vi "Z to circle.vi"(8 "Error In":errorcluster, 10 "Plot points":i32=90, 11 "Z":cdb[](array[numeric])) -> (0 "Error Out":errorcluster, 1 "y0":dbl, 2 "x0":dbl, 3 "plot":cluster{"Array":dbl[], "Array":dbl[]}, 4 "r":dbl format="%.2f", 5 "theta":dbl, 6 "Circle fit":cluster{"Array":dbl[], "Array":dbl[]}[](graph))   [LabVIEW 2016]
uses:
  <vilib>/gmath/NI_Gmath.lvlib
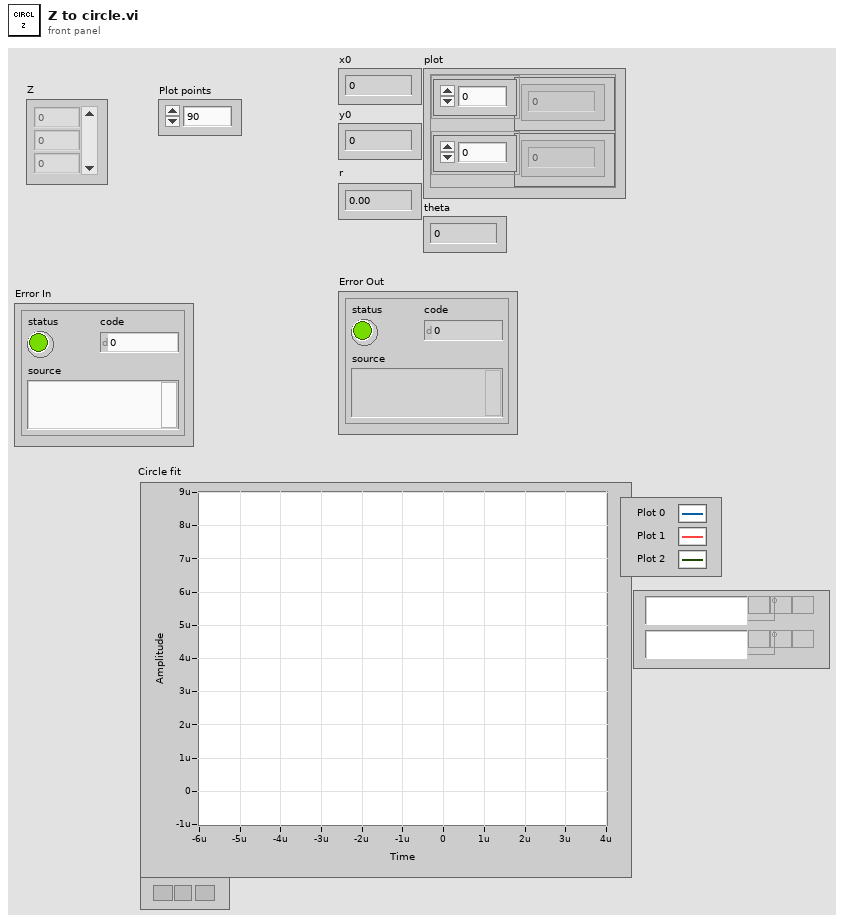
[diagram p1: front panel]
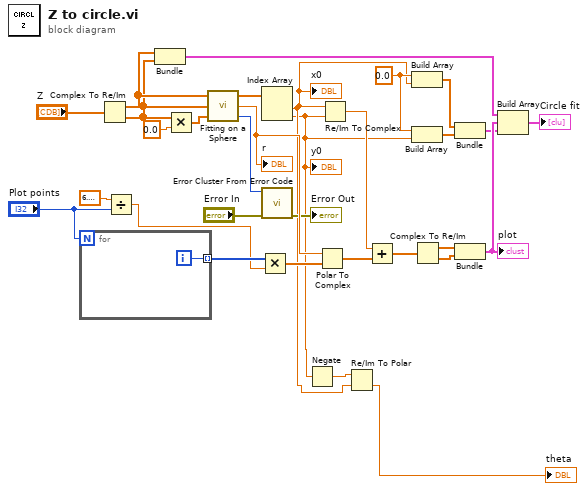
[diagram p0: block diagram]
diagram:
  w6 = 0.0
  n1 = for {
    N: "Plot points" -> [_]
    tunnel: [w32] -> w29 mode=indexing
    i -> [w32]
  }
  n2 = Complex To Re/Im(x + iy="Z") -> (x=w12:dbl[], y=w11:dbl[])
  n3 = Divide(x=6.283185307179586, y="Plot points") -> (x/y=w26:dbl)
  n4 = Bundle(w12, w11) -> (w10:cluster{dbl[], dbl[]})  [unwired: 1 in]
  n5 = Multiply(x=w11, y=0.0) -> (x*y=w31:dbl[])
  n6 = call <vilib>:"Fitting on a Sphere.vi"("Z"=w31, "Y"=w11, "X"=w12) -> ("error"=w17:i32, "r"=w24:dbl, "x0, y0, z0"=w23:dbl[])
  "r" <- w24
  n7 = Multiply(x=w29, y=w26) -> (x*y=w25:dbl[])
  n8 = Index Array(array=w23) -> (element #1=w3:dbl, element #2=w2:dbl)  [unwired: 2 in]
  "x0" <- w3
  "y0" <- w2
  n9 = call <vilib>:"Error Cluster From Error Code.vi"("error in (no error)"="Error In", "error code (0)"=w17) -> ("error out"=→"Error Out":errorcluster)  [unwired: 7 in]
  n10 = Negate(x=w2) -> (-x=w1:dbl)
  n11 = Polar To Complex(1:w25, 2:w24) -> (0:w22:cdb[])
  n12 = Re/Im To Complex(1:w2, 2:w3) -> (0:w14:cdb)
  n13 = Re/Im To Polar(2:w3, 3:w1) -> (0:→"theta":dbl)  [unwired: 1 out]
  n14 = Add(x=w14, y=w22) -> (x+y=w21:cdb[])
  n15 = Build Array(w6, w3) -> (w7:dbl[])
  n16 = Build Array(w6, w2) -> (w8:dbl[])
  n17 = Complex To Re/Im(x + iy=w21) -> (x=w20:dbl[], y=w19:dbl[])
  n18 = Bundle(w7, w8) -> (w5:cluster{dbl[], dbl[]})  [unwired: 1 in]
  n19 = Bundle(w20, w19) -> (w9:cluster{dbl[], dbl[]})  [unwired: 1 in]
  "plot" <- w9
  n20 = Build Array(w10, w9, w5) -> (→"Circle fit":cluster{dbl[], dbl[]}[])
